vi "switch_data.vi"() -> ()   [LabVIEW 2014]
uses:
  <vilib>/wsapi/Web Request.lvclass
  DataManager/StateStore/Controls/DataFunction.ctl
panel:
  in  "LabVIEW Web Service Request 2":refnum<class "Web Request.lvclass">
  # "Use the Web Service Request input terminal to call the VIs on the Web Services palette. Do not remove it from the connector pane unless you don't need access to the palette."
  # "Each additional control wired to the connector pane will be available as an input in the URL. To include an indicator in terminal-mode output (the default setting), it must also be wired to the connector pane."
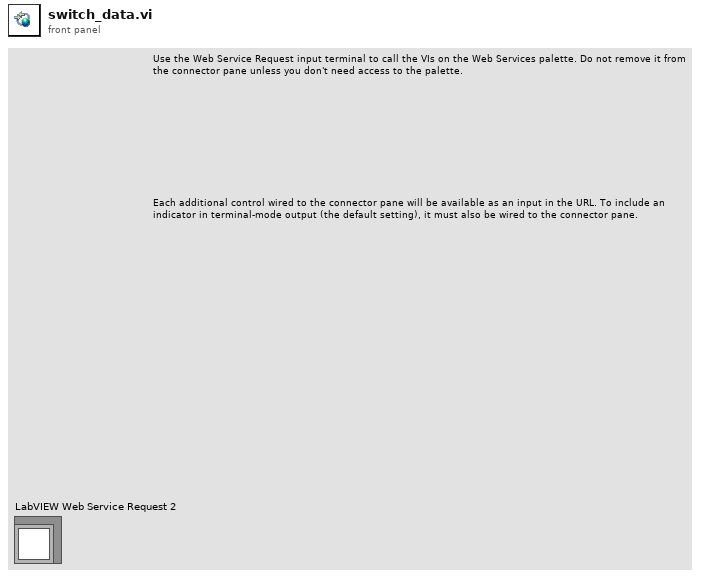
[diagram p1: front panel]
types:
  T1 = cluster{"switch_posit":cluster{"x":dbl, "y":dbl, "z":dbl}, "manual":bool}
  T2 = typedef "DataFunction.ctl" = enum16{"Initialise", "Release", "Get Data", "Set Data", "Preview Data"}
  T3 = typedef "CData Core Control.ctl" = cluster{"train_data_array":cluster{"uuid":string, "int":i32, "posit_array":cluster{"x":dbl, "y":dbl, "z":dbl}[]}[], "train_control_array":cluster{"uuid":string, "throttle":dbl, "brake":dbl, "horn":dbl, "wait":dbl, "name":string, "mode":string, "dest":string}[], "switch_data_array":cluster{"switch_posit":cluster{"x":dbl, "y":dbl, "z":dbl}, "manual":bool}[], "switch_control_array":cluster{"switch_posit":cluster{"x":dbl, "y":dbl, "z":dbl}, "switch":bool, "invert":bool, "wait":dbl}[]}
  T4 = cluster{"switch_posit":cluster{"x":dbl, "y":dbl, "z":dbl}, "switch":bool, "invert":bool, "wait":dbl}[]
  T5 = cluster{"switch_posit":cluster{"x":dbl, "y":dbl, "z":dbl}, "manual":bool}[]
  T6 = cluster{"switch_posit":cluster{"x":dbl, "y":dbl, "z":dbl}, "switch":bool, "invert":bool, "wait":dbl}
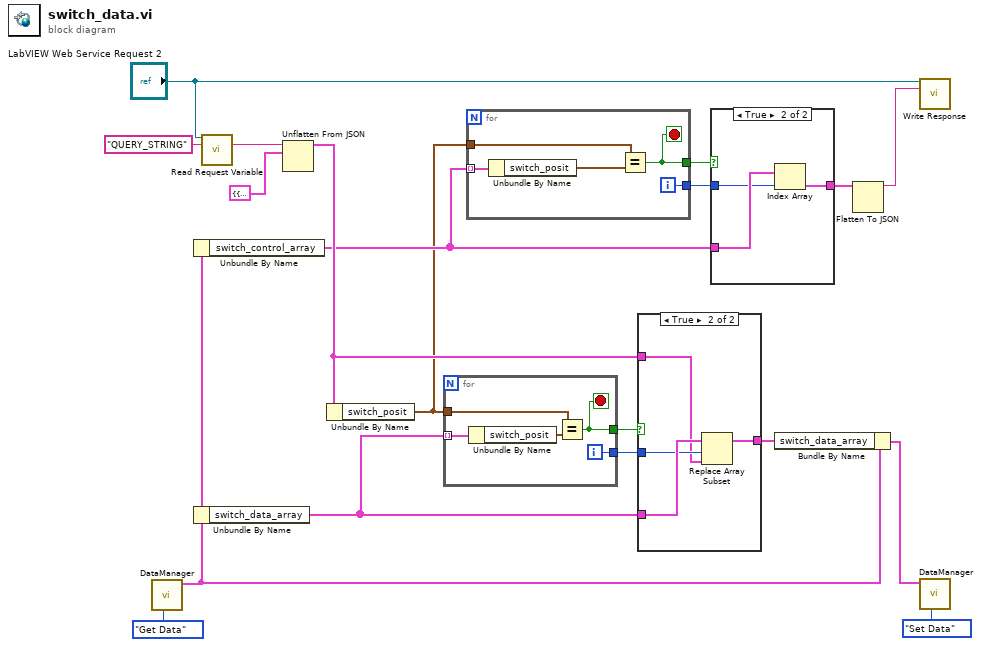
[diagram p0: block diagram]
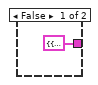
[diagram p2: hidden frame]
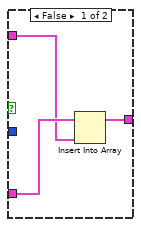
[diagram p3: hidden frame]
diagram:
  n1 = call "DataManager.vi"("DataFunction"=DataFunction."Get Data") -> ("CData Out"=w1:T3)  [unwired: 9 in, 1 out]
  n2 = Unbundle By Name(w1) -> ("switch_control_array"=w8:T4)
  n3 = Unbundle By Name(w1) -> ("switch_data_array"=w14:T5)
  n4 = call <vilib>:"Read Request Variable.vi"("LabVIEW Web Service Request"="LabVIEW Web Service Request 2", "variable name"="QUERY_STRING") -> ("value"=w3:string)  [unwired: 11 in, 2 out]
  n5 = Unflatten From JSON(JSON string=w3, type and defaults=T1 {"switch_posit"={"x"=0.0, "y"=0.0, "z"=0.0}, "manual"=FALSE} ("switch_data")) -> (value=w13:T1)  [unwired: 5 in, 1 out]
  n6 = Unbundle By Name(w13) -> ("switch_posit"=w2:cluster{"x":dbl, "y":dbl, "z":dbl})
  n7 = for {
    tunnel: w14 -> [w24] mode=indexing
    tunnel: w2 -> [w22]
    tunnel: [w21] -> w16
    tunnel: [w20] -> w15
    i -> [w20]
    stop <- w21 stop-if-true
    n8 = Unbundle By Name(w24) -> ("switch_posit"=w23:cluster{"x":dbl, "y":dbl, "z":dbl})
    n9 = Equal?(x=w22, y=w23) -> (x = y?=w21:bool)
  }
  n10 = for {
    tunnel: w8 -> [w29] mode=indexing
    tunnel: w2 -> [w28]
    tunnel: [w27] -> w10
    tunnel: [w26] -> w9
    i -> [w26]
    stop <- w27 stop-if-true
    n11 = Unbundle By Name(w29) -> ("switch_posit"=w25:cluster{"x":dbl, "y":dbl, "z":dbl})
    n12 = Equal?(x=w28, y=w25) -> (x = y?=w27:bool)
  }
  n13 = case shown="True" w16 {
    tunnel: w15 -> [_ w35]
    tunnel: w14 -> [w32 w36]
    tunnel: w13 -> [w31 w34]
    tunnel: [w30 w33] -> w12
    frame False {
      n14 = Insert Into Array(array=w32, new element=w31) -> (w30:T5)  [unwired: 1 in]
    }
    frame True {
      n15 = Replace Array Subset(array=w36, new element=w34, index=w35) -> (w33:T5)
    }
  }
  n16 = case shown="True" w10 {
    tunnel: w9 -> [_ w39]
    tunnel: w8 -> [_ w40]
    tunnel: [T6 {"switch_posit"={"x"=0.0, "y"=0.0, "z"=0.0}, "switch"=FALSE, "invert"=FALSE, "wait"=0.0} ("switch_control") w38] -> w6
    frame False {
    }
    frame True {
      n17 = Index Array(array=w40, index=w39) -> (element=w38:T6)
    }
  }
  n18 = Bundle By Name(cluster=w1, "switch_data_array"=w12) -> (w17:T3)
  n19 = Flatten To JSON(anything=w6) -> (JSON string=w5:string)  [unwired: 2 in, 1 out]
  n20 = call <vilib>:"Write Response.vi"("LabVIEW Web Service Request"="LabVIEW Web Service Request 2", "response string"=w5) -> ()  [unwired: 12 in, 2 out]
  n21 = call "DataManager.vi"("DataFunction"=DataFunction."Set Data", "CData In"=w17) -> ()  [unwired: 8 in, 2 out]
